vi "wait.vi"(8 "error in (no error)":errorcluster, 11 "DL090130ExperimentController in":refnum<class "ExperimentControllerDL090130Interval.lvclass">) -> (0 "error out":errorcluster, 3 "DL090130ExperimentController out":refnum<class "ExperimentControllerDL090130Interval.lvclass">)   [LabVIEW 2010, in "ExperimentControllerDL090130Interval.lvclass"]
uses:
  ExperimentControllerDL090130Interval.lvclass
  schedule_entry_cluster.ctl
  internal_trigger_enum.ctl
  ExperimentControllerDL090130Interval.lvclass/ExperimentControllerDL090130Interval.ctl
  Sweep/GenericSweep/GenericSweep/GenericSweep.lvclass
  GenericExperimentController/GenericExperimentController/trigger_enum.ctl
  common/classes/ErrorController/ErrorController/class_data.vi
  GenericExperimentController/GenericExperimentController/GenericExperimentController.lvclass
  common/classes/ErrorController/ErrorController/ErrorController.lvclass
panel:
  out "x >= y?":bool
  out "appended array":T1[](array[typedef])
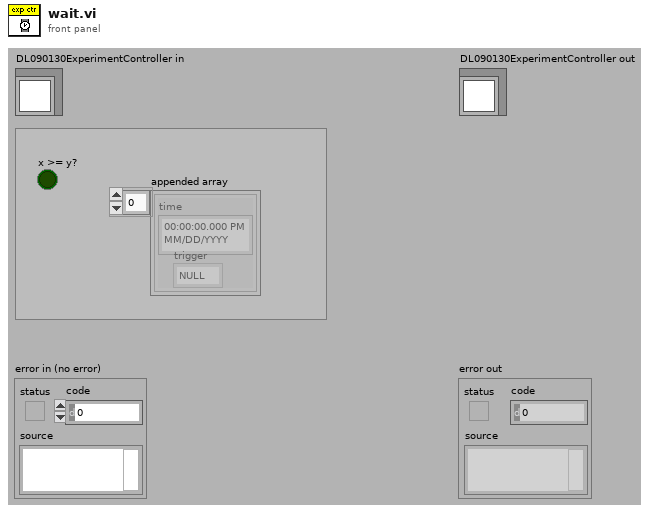
[diagram p1: front panel]
types:
  T1 = typedef "ExperimentControllerDL090130Interval.lvclass/schedule_entry_cluster.ctl" = cluster{"time":timestamp, "trigger":T2}
  T2 = typedef "ExperimentControllerDL090130Interval.lvclass/internal_trigger_enum.ctl" = enum16{"NULL", "initialise", "terminate", "start", "stop", "proceed", "prepare", "start sweep"}
  T3 = typedef "GenericExperimentController.lvclass/trigger_enum.ctl" = enum16{"NULL", "proceed", "prepare"}
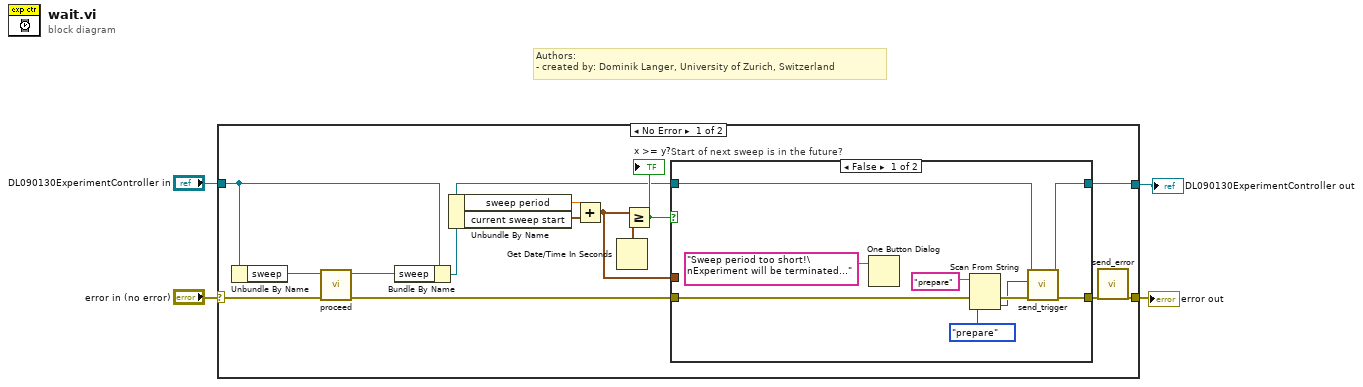
[diagram p0: block diagram]
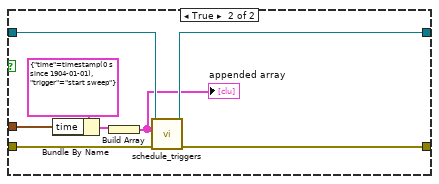
[diagram p2: hidden frame]
diagram:
  # "Authors: \n- created by: Dominik Langer, University of Zurich, Switzerland"
  n1 = case shown="No Error" "error in (no error)" {
    selector: "error in (no error)" -> [w10 w37]
    tunnel: [w6 w37] -> w3
    tunnel: [w15 w36] -> w1
    tunnel: "DL090130ExperimentController in" -> [w12 w36]
    frame No Error {
      n2 = Unbundle By Name(w12) -> ("sweep"=w8:refnum<class "GenericSweep.lvclass">)
      n3 = call-dynamic "proceed.vi"("error in (no error)"=w10, "GenericSweep in"=w8) -> ("error out"=w9:errorcluster, "GenericSweep out"=w7:refnum<class "GenericSweep.lvclass">)  [unwired: 8 in]
      n4 = Bundle By Name(cluster=w12, "sweep"=w7) -> (w11:refnum<class "ExperimentControllerDL090130Interval.lvclass">)
      n5 = Unbundle By Name(w11) -> ("sweep period"=w18:dbl[unit], "current sweep start"=w17:timestamp)
      n6 = Add(x=w18, y=w17) -> (x+y=w14:timestamp)
      n7 = Get Date/Time In Seconds() -> (seconds since 1Jan1904=w16:timestamp)
      n8 = Greater Or Equal?(x=w14, y=w16) -> (x >= y?=w13:bool)
      "x >= y?" <- w13
      n9 = case "Start of next sweep is in the future?" shown="False" w13 {
        tunnel: w9 -> [w22 w35]
        tunnel: [w27 w34] -> w5
        tunnel: w11 -> [w26 w33]
        tunnel: [w25 w32] -> w15
        tunnel: w14 -> [_ w31]
        frame False {
          n10 = One Button Dialog(message="Sweep period too short!\nExperiment will be terminated...") -> ()  [unwired: 2 out]
          n11 = Scan From String(input string="prepare", error in=w22, default 1=trigger_enum."prepare" ("trigger")) -> (error out=w21:errorcluster, output 1=w19:T3)  [unwired: 2 in, 2 out]
          n12 = call-dynamic "send_trigger.vi"("error in (no error)"=w21, "trigger"=w19, "GenericExperiment in"=w26) -> ("error out"=w27:errorcluster, "GenericExperiment out"=w25:refnum<class "ExperimentControllerDL090130Interval.lvclass">)  [unwired: 7 out]
        }
        frame True {
          n13 = Bundle By Name(cluster=T1 {"time"=timestamp(0 s since 1904-01-01), "trigger"=enum."start sweep"} ("schedule entry"), "time"=w31) -> (w28:T1)
          n14 = Build Array(w28) -> (w29:T1[])
          "appended array" <- w29
          n15 = call-dynamic "schedule_triggers.vi"("error in (no error)"=w35, "new schedule entries"=w29, "DL090130ExperimentController in"=w33) -> ("error out"=w34:errorcluster, "DL090130ExperimentController out"=w32:refnum<class "ExperimentControllerDL090130Interval.lvclass">)  [unwired: 7 out]
        }
      }
      n16 = call "send_error.vi"("error in (no error)"=w5) -> ("error out"=w6:errorcluster)  [unwired: 10 in]
    }
    frame Error {
    }
  }
  "error out" <- w3
  "DL090130ExperimentController out" <- w1
